vi "MultiTest Status.vi"(0 "numTrip":i32[](array[numeric]), 1 "Period":u8, 2 "KTu":dbl[](array[numeric]), 3 "KG20":dbl[](array[numeric]), 4 "temperature":dbl[](array[numeric])) -> (5 "Status":string[][](array[string]))   [LabVIEW 2015]
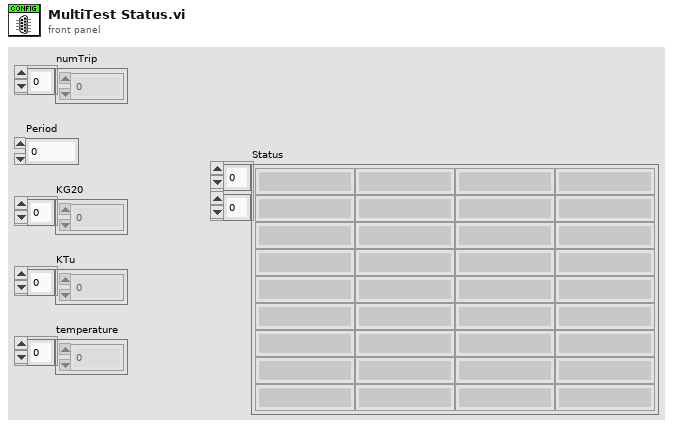
[diagram p1: front panel]
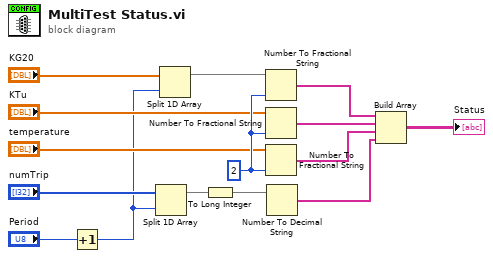
[diagram p0: block diagram]
diagram:
  w9 = i16 2 ("precision (6)")
  n1 = Increment(x="Period") -> (x+1=w1:u8)
  n2 = Split 1D Array(array="numTrip", index=w1) -> (first subarray=w13:i32[])  [unwired: 1 out]
  n3 = Split 1D Array(array="KG20", index=w1) -> (first subarray=w11:dbl[])  [unwired: 1 out]
  n4 = To Long Integer(number=w13) -> (32bit integer=w5:i32[])
  n5 = Number To Fractional String(number=w11, precision (6)=w9) -> (F-format string=w6:string[])  [unwired: 2 in]
  n6 = Number To Fractional String(number="KTu", precision (6)=w9) -> (F-format string=w7:string[])  [unwired: 2 in]
  n7 = Number To Fractional String(number="temperature", precision (6)=w9) -> (F-format string=w8:string[])  [unwired: 2 in]
  n8 = Number To Decimal String(number=w5) -> (decimal integer string=w14:string[])  [unwired: 1 in]
  n9 = Build Array(w6, w7, w8, w14) -> (→"Status":string[][])
